vi "Change Detect Boolean.vi"(1 "In":bool) -> (0 "Changed?":bool)   [LabVIEW 2015]
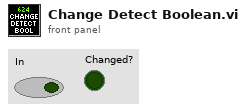
[diagram p1: front panel]
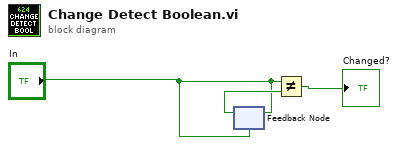
[diagram p0: block diagram]
diagram:
  n1 = feedback-in #1("In") -> ()
  n2 = feedback #1("In") -> (w3:bool)
  n3 = Not Equal?(x="In", y=w3) -> (x != y?=→"Changed?":bool)
